vi "Windows SYSTEMTIME to String.vi"(1 "time format string (%c)":string="%c", 2 "UTC Date and Time in":T1={"Year"=0, "Month"=1, "DayOfWeek"=0, "Day"=0, "Hour"=0, "Minute"=0, "Seconds"=0, "Milliseconds"=0} {"DayOfWeek" items=["Sunday", "Monday", "Tuesday", "Wednesday", "Thursday", "Friday", "Saturday"]; "Month" items=["", "January", "February", "March", "April", "May", "June", "July", "August", "September", "October", "November", "December"]}) -> (0 "UTC Date and Time out (string)":string)   [LabVIEW 2019, in "TSC Event Logger.lvlib" / "Log Sinks.lvclass"]
doc: "This VI takes in a Windows SYSTEMTIME structure and displays the date and time in seconds since 12:00 a.m., January 1, 1904, Universal time, in a format you specify.\n\nThe SYSTEMTIME structure consists of:\n<B>Year</B>\nSpecifies the current year.\n<B>Month</B>\nSpecifies the current month; January = 1, February = 2, and so on.\n<B>DayOfWeek</B>\nSpecifies the current day of the week; Sunday = 0, Monday = 1, and so on.\n<B>Day</B>\nSpecifies the current day of the month.\n<B>Hour</B>\nSpecifies the current hour.\n<B>Minute</B>\nSpecifies the current minute.\n<B>Second</B>\nSpecifies the current second.\n<B>Milliseconds</B>\nSpecifies the current millisecond.\n\nAdapted from Ed Dickens:\nhttps://forums.ni.com/t5/LabVIEW/file-date-created/m-p/109838/highlight/true?profile.language=en#M66474\n\nThe <B>time format string</B> can contain any combination of the following codes: %H (hour, 24-hour clock), %I (hour, 12-hour clock), %M (minute), %S (second), %p (a.m./p.m. flag), %d (day of month), %m (month number), %y (year within century), %Y (year including century), %a (abbreviated weekday name), %x (locale-specific date), %X (locale-specific time), %c (locale-specific date/time), %<digit>u (fractional seconds with <digit> precision)."
uses:
  Log Sinks.lvclass
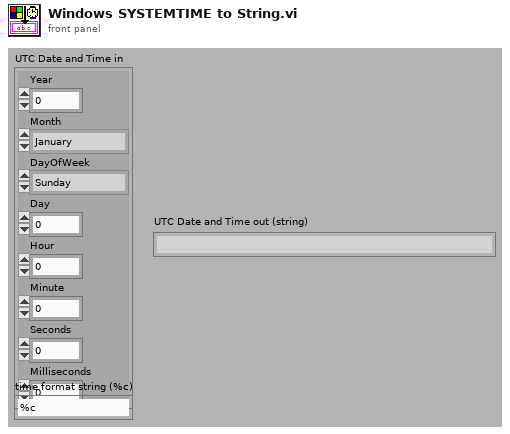
[diagram p1: front panel]
types:
  T1 = cluster{"Year":u16, "Month":u16, "DayOfWeek":u16, "Day":u16, "Hour":u16, "Minute":u16, "Seconds":u16, "Milliseconds":u16}
  T2 = cluster{"Seconds":i32, "Minute":i32, "Hour":i32, "Day":i32, "Month":i32, "Year":i32, "DayOfWeek":i32, i32, i32}
  T3 = cluster{"Year":i32, "Month":i32, "DayOfWeek":i32, "Day":i32, "Hour":i32, "Minute":i32, "Seconds":i32, "Milliseconds":i32}
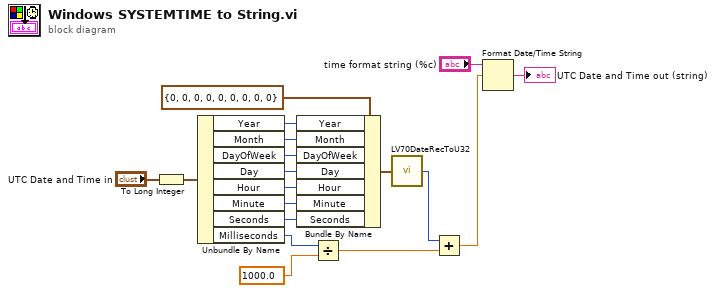
[diagram p0: block diagram]
diagram:
  n1 = To Long Integer(number="UTC Date and Time in") -> (32bit integer=w17:T3)
  n2 = Unbundle By Name(w17) -> ("Year"=w15:i32, "Month"=w9:i32, "DayOfWeek"=w11:i32, "Day"=w10:i32, "Hour"=w12:i32, "Minute"=w13:i32, "Seconds"=w14:i32, "Milliseconds"=w7:i32)
  n3 = Bundle By Name(cluster=T2 {"Seconds"=0, "Minute"=0, "Hour"=0, "Day"=0, "Month"=0, "Year"=0, "DayOfWeek"=0, 0, 0} ("output cluster"), "Year"=w15, "Month"=w9, "DayOfWeek"=w11, "Day"=w10, "Hour"=w12, "Minute"=w13, "Seconds"=w14) -> (w8:T2)
  n4 = Divide(x=w7, y=1000.0) -> (x/y=w4:dbl)
  n5 = call <vilib>:"LV70DateRecToU32.vi"("date time rec"=w8) -> ("Time"=w5:u32)
  n6 = Add(x=w5, y=w4) -> (x+y=w3:dbl)
  n7 = Format Date/Time String(time format string (%c)="time format string (%c)", seconds (now)=w3) -> (date/time string=→"UTC Date and Time out (string)":string)  [unwired: 1 in]
